vi "PH_BeamlineInformation.PC _Head_in_Use.vi"(0 "i ref in":refnum<vi>, 2 "In Use Service Name":string, 3 "In Use?":bool, 4 "no link?":bool, 5 "error in (no error)":errorcluster) -> (14 "i ref out":refnum<vi>, 19 "error out":errorcluster)   [LabVIEW 2014, in "PH_BeamlineInformation.lvlib"]
doc: "This VI writes the in Use information of the related PU to own attributes and the GUI elements."
uses:
  PH_BeamlineInformation.lvlib
  PH_Basics/PH_Common/PH_Common.lvlib
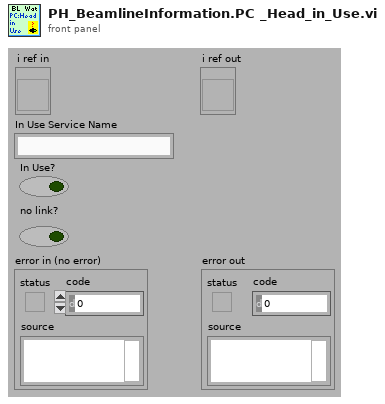
[diagram p1: front panel]
types:
  T1 = typedef "PH_BeamlineInformation.lvlib/PH_BeamlineInformation.i attribute.ctl" = cluster{"BL GUI Elements of Services":cluster{"Service Name":string, "GUI Elements":refnum<vi>[], "Status":i32}[], "Powermeters":T2, "Efficiency":T3, "Heads":T4[]}
  T2 = typedef "PH_BeamlineInformation.lvlib/PH_BeamlineInformation.Powermeter.ctl" = cluster{"ns FE":cluster{"GUI Ref":refnum<vi>, "Value":dbl}, "fs FE":cluster{"GUI Ref":refnum<vi>, "Value":dbl}, "PA":cluster{"GUI Ref":refnum<vi>, "Value":dbl}, "MA":cluster{"GUI Ref":refnum<vi>, "Value":dbl}, "Z6 green":cluster{"GUI Ref":refnum<vi>, "Value":dbl}, "Z6 IR":cluster{"GUI Ref":refnum<vi>, "Value":dbl}, "Z6 COS":cluster{"GUI Ref":refnum<vi>, "Value":dbl}}
  T3 = typedef "PH_BeamlineInformation.lvlib/PH_BeamlineInformation.Efficiency.ctl" = cluster{"PA Gain":cluster{"GUI Ref":refnum<vi>, "Value":dbl}, "MA Gain":cluster{"GUI Ref":refnum<vi>, "Value":dbl}, "Z6 green Conversion":cluster{"GUI Ref":refnum<vi>, "Value":dbl}, "Z6 Comp Losses":cluster{"GUI Ref":refnum<vi>, "Value":dbl}}
  T4 = typedef "PH_BeamlineInformation.lvlib/PH_BeamlineInformation.Head.ctl" = cluster{"PowerUnit":T5, "in use":cluster{"Value":bool, "GUI Ref":refnum<vi>, "linked":bool}, "voltage":cluster{"Value":dbl, "GUI Ref":refnum<vi>, "linked":bool}}
  T5 = typedef "PH_PP_Common.lvlib/PH_PP_Common.PUs.ctl" = enum16{"no Info", "PA-19mm-1", "PA-19mm-2", "PA-45mm-PILC", "PA-45mm-MAIN", "MA-PU-1", "MA-PU-2", "MA-PU-3", "MA-PU-4", "MA-PU-5", "MA-PU-6", "MA-FR", "MA-PILC", "PA-45mm-DP"}
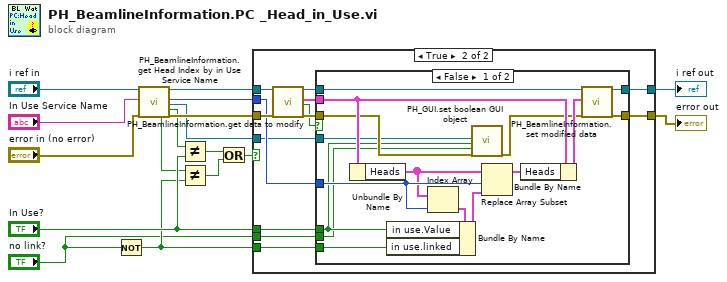
[diagram p0: block diagram]
diagram:
  n1 = Not(x="no link?") -> (.not. x?=w6:bool)
  n2 = call "PH_BeamlineInformation.get Head Index by in Use Service Name.vi"("i ref in"="i ref in", "In Use Service Name"="In Use Service Name", "error in (no error)"="error in (no error)") -> ("current in use linked?"=w7:bool, "i ref out"=w12:refnum<vi>, "index of element"=w10:i32, "in Use GUI Ref"=w3:refnum<vi>, "current in use value"=w14:bool, "error out"=w15:errorcluster)  [unwired: 11 in]
  n3 = Not Equal?(x=w14, y="In Use?") -> (x != y?=w13:bool)
  n4 = Not Equal?(x=w7, y=w6) -> (x != y?=w4:bool)
  n5 = Or(x=w13, y=w4) -> (x .or. y?=w5:bool)
  n6 = case shown="True" w5 {
    tunnel: w15 -> [w19 w32]
    tunnel: "In Use?" -> [_ w31]
    tunnel: [w19 w29] -> w2
    tunnel: w12 -> [w18 w28]
    tunnel: [w18 w26] -> w11
    tunnel: w10 -> [_ w23]
    tunnel: w6 -> [_ w22]
    tunnel: w3 -> [_ w21]
    tunnel: "no link?" -> [_ w20]
    frame False {
    }
    frame True {
      n7 = call "PH_BeamlineInformation.get data to modify.vi"("i ref in"=w28, "error in (no error)"=w32) -> ("i ref out"=w27:refnum<vi>, "i attribute"=w25:T1, "timed out"=w24:bool, "error out"=w30:errorcluster)  [unwired: 14 in]
      n8 = case shown="False" w24 {
        tunnel: w31 -> [w34 _]
        tunnel: w30 -> [w37 w49]
        tunnel: [w48 w49] -> w29
        tunnel: w27 -> [w47 w50]
        tunnel: [w46 w50] -> w26
        tunnel: w25 -> [w44 _]
        tunnel: w23 -> [w41 _]
        tunnel: w22 -> [w38 _]
        tunnel: w21 -> [w35 _]
        tunnel: w20 -> [w33 _]
        frame False {
          n9 = Unbundle By Name(w44) -> ("Heads"=w40:T4[])
          n10 = Index Array(array=w40, index=w41) -> (element=w43:T4)
          n11 = Bundle By Name(cluster=w43, "in use.Value"=w34, "in use.linked"=w38) -> (w42:T4)
          n12 = call "PH_GUI.set boolean GUI object.vi"("Boolean Knob GUI Ref"=w35, "Value"=w34, "Blinking? (false)"=w33, "error in (no error)"=w37) -> ("error out"=w36:errorcluster)  [unwired: 15 in]
          n13 = Replace Array Subset(array=w40, new element=w42, index=w41) -> (w39:T4[])
          n14 = Bundle By Name(cluster=w44, "Heads"=w39) -> (w45:T1)
          n15 = call "PH_BeamlineInformation.set modified data.vi"("i ref in"=w47, "i attribute"=w45, "error in (no error)"=w36) -> ("i ref out"=w46:refnum<vi>, "error out"=w48:errorcluster)  [unwired: 15 in]
        }
        frame True {
        }
      }
    }
  }
  "error out" <- w2
  "i ref out" <- w11
